vi "解包属性.vi"(0 "测试数据输入":T1, 5 "数据属性":variant, 11 "错误输入（无错误）":errorcluster) -> (4 "测试数据输出":T1, 15 "错误输出":errorcluster)   [LabVIEW 2020]
uses:
  <vilib>/NI/Tools/String/Tools_String.lvlib
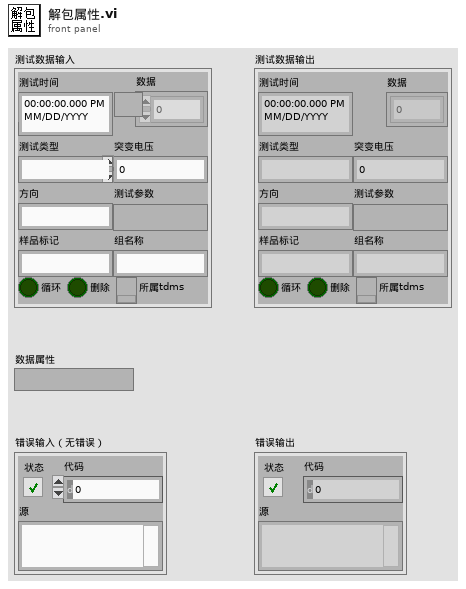
[diagram p1: front panel]
types:
  T1 = typedef "测试数据类型.ctl" = cluster{"测试时间":timestamp, "数据":dbl[][], "测试类型":string, "方向":string, "样品标记":string, "突变电压":i32, "测试参数":variant, "循环":bool, "删除":bool, "组名称":string, "所属tdms":refnum<k34>}
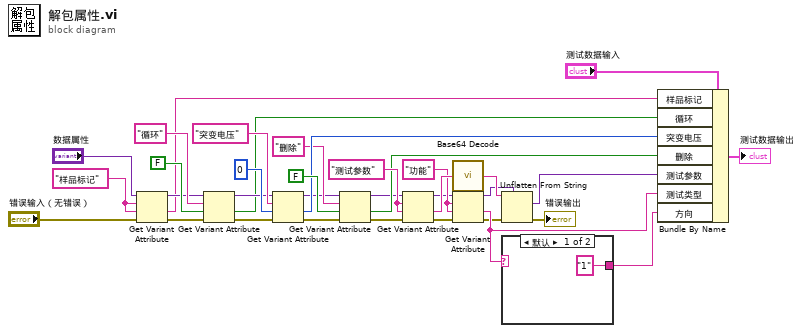
[diagram p0: block diagram]
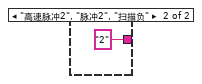
[diagram p2: hidden frame]
diagram:
  w32 = "测试参数" ("名称")
  w28 = "样品标记" ("名称")
  w18 = "功能" ("名称")
  n1 = Get Variant Attribute(Variant="数据属性", name=w28, default value (empty Variant)=w28, error in="错误输入（无错误）") -> (duplicate Variant=w23:variant, value=w21:string, error out=w29:errorcluster)  [unwired: 1 out]
  n2 = Get Variant Attribute(Variant=w23, name="循环" ("名称"), default value (empty Variant)=FALSE, error in=w29) -> (duplicate Variant=w22:variant, value=w20:bool, error out=w30:errorcluster)  [unwired: 1 out]
  n3 = Get Variant Attribute(Variant=w22, name="突变电压" ("名称"), default value (empty Variant)=0, error in=w30) -> (duplicate Variant=w13:variant, value=w19:i32, error out=w12:errorcluster)  [unwired: 1 out]
  n4 = Get Variant Attribute(Variant=w13, name="删除" ("名称"), default value (empty Variant)=FALSE, error in=w12) -> (duplicate Variant=w8:variant, value=w14:bool, error out=w7:errorcluster)  [unwired: 1 out]
  n5 = Get Variant Attribute(Variant=w8, name=w32, default value (empty Variant)=w32, error in=w7) -> (duplicate Variant=w10:variant, value=w33:string, error out=w9:errorcluster)  [unwired: 1 out]
  n6 = call <vilib>:"Base64 Decode.vi"("base64 string"=w33) -> ("normal string"=w11:string)
  n7 = Get Variant Attribute(Variant=w10, name=w18, default value (empty Variant)=w18, error in=w9) -> (duplicate Variant=w3:variant, value=w5:string, error out=w2:errorcluster)  [unwired: 1 out]
  n8 = Unflatten From String(type=w3, binary string=w11, error in (no error)=w2) -> (value=w4:variant, error out=→"错误输出":errorcluster)  [unwired: 2 in, 1 out]
  n9 = case shown="默认" w5 {
    tunnel: ["1" ("名称") "2" ("名称")] -> w6
    frame Default {
    }
    frame "高速脉冲2", "脉冲2", "扫描负" {
    }
  }
  n10 = Bundle By Name(cluster="测试数据输入", "样品标记"=w21, "循环"=w20, "突变电压"=w19, "删除"=w14, "测试参数"=w4, "测试类型"=w5, "方向"=w6) -> (→"测试数据输出":T1)
